vi "Enable Output.vi"(7 "Chanel":string, 9 "ON/OFF":bool, 11 "VISA Source":string) -> (4 "error out":errorcluster)   [LabVIEW 2020]
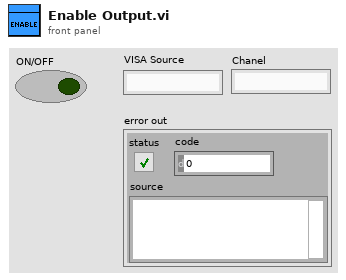
[diagram p1: front panel]
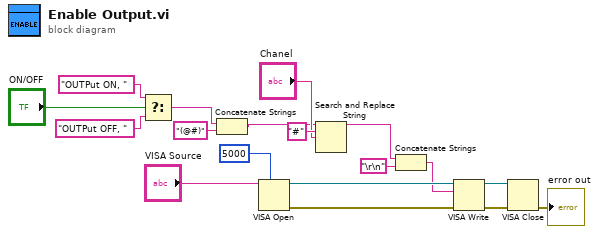
[diagram p0: block diagram]
diagram:
  n1 = Select(t="OUTPut ON, " ("string"), s="ON/OFF", f="OUTPut OFF, " ("string")) -> (s? t:f=w2:string)
  n2 = Concatenate Strings(w2, "(@#)" ("string")) -> (w8:string)
  n3 = VISA Open(timeout (0)=u32 5000 ("VISA Open timeout (0)"), VISA resource name="VISA Source") -> (VISA resource name=w18:refnum<visa-resource-name>, error out=w17:errorcluster)  [unwired: 3 in]
  n4 = Search and Replace String(input string=w8, search string="#", replace string="Chanel") -> (result string=w7:string)  [unwired: 5 in, 3 out]
  n5 = Concatenate Strings(w7, "\r\n") -> (w12:string)
  n6 = VISA Write(VISA resource name=w18, write buffer=w12, error in (no error)=w17) -> (VISA resource name out=w15:refnum<visa-resource-name>, error out=w14:errorcluster)  [unwired: 1 out]
  n7 = VISA Close(VISA resource name=w15, error in (no error)=w14) -> (error out=→"error out":errorcluster)
